vi "ModemTelemetryDecode.vi"(8 "Error In":errorcluster, 11 "Encoded Data":u8[](array[numeric])) -> (0 "Error Out":errorcluster, 3 "TelemetryPacket":T1)   [LabVIEW 2010]
uses:
  ModemTelemetryPacket.ctl
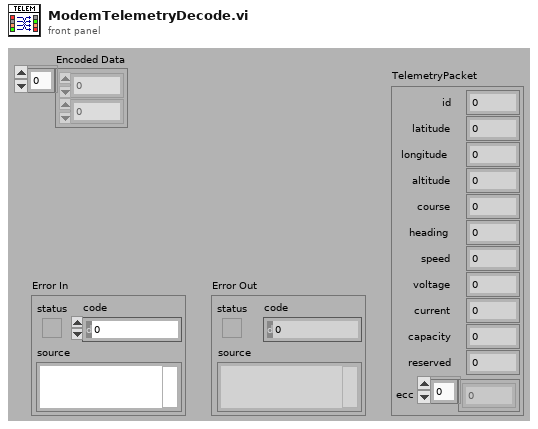
[diagram p1: front panel]
types:
  T1 = typedef "ModemTelemetryPacket.ctl" = cluster{"id":u16, "latitude":i32, "longitude":i32, "altitude":i16, "course":i16, "heading":i16, "speed":i16, "voltage":u8, "current":u8, "capacity":u16, "reserved":u16, "ecc":u8[]}
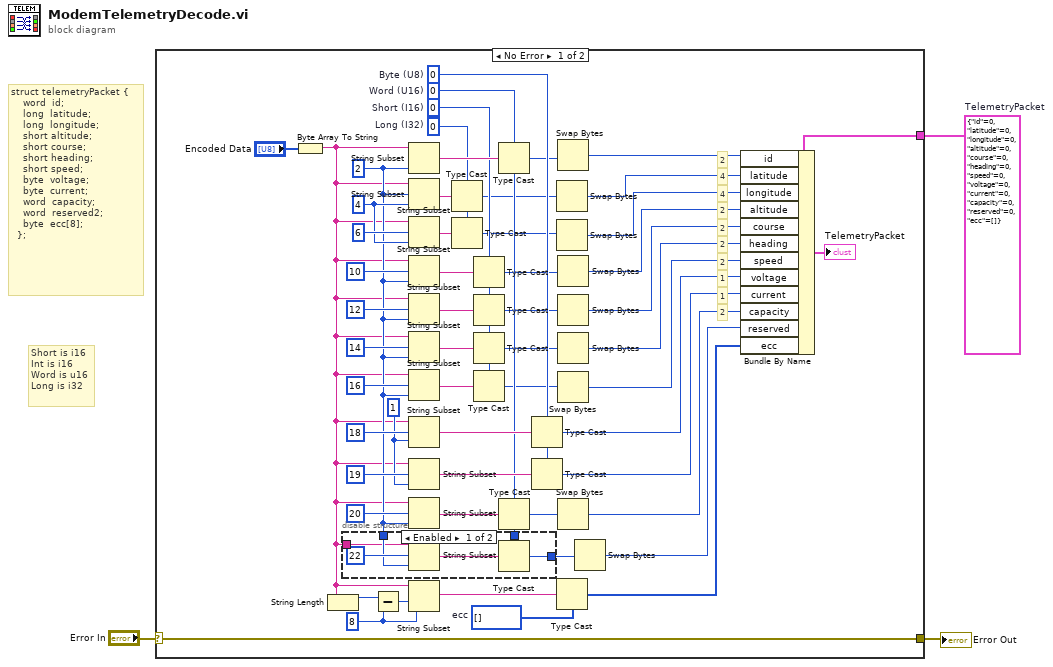
[diagram p0: block diagram]
diagram:
  w1 = T1 {"id"=0, "latitude"=0, "longitude"=0, "altitude"=0, "course"=0, "heading"=0, "speed"=0, "voltage"=0, "current"=0, "capacity"=0, "reserved"=0, "ecc"=[]}  # TelemetryPacket
  # "struct telemetryPacket {\n    word  id;\n    long  latitude;\n    long  longitude;\n    short altitude;\n    short course;\n    short heading;\n    short speed;\n    byte  voltage;\n    byte  current;\n    word  capacity;\n    word  reserved2;\n    byte  ecc[8];\n  };"
  # "Short is i16\nInt is i16\nWord is u16\nLong is i32"
  n1 = case shown="No Error" "Error In" {
    selector: "Error In" -> [w59 w66]
    tunnel: [w59 w66] -> w2
    tunnel: w1 -> [w57 _]
    frame No Error {
      w22 = u16 0  # Word (U16)
      w24 = 8 ("length (rest)")
      w29 = u8[] []  # ecc
      w36 = 1 ("length (rest)")
      w37 = u8 0  # Byte (U8)
      w52 = 0  # Long (I32)
      w49 = 4 ("length (rest)")
      w23 = i16 0  # Short (I16)
      w31 = 2 ("length (rest)")
      # "2"
      # "1"
      # "1"
      # "2"
      # "2"
      # "2"
      # "2"
      # "4"
      # "4"
      # "2"
      n2 = Byte Array To String(unsigned byte array="Encoded Data") -> (string=w27:string)
      n3 = String Length(string=w27) -> (length=w26:i32)
      n4 = disable-structure shown="Enabled" {
        disable-tunnel: w31 -> [w64 _]
        disable-tunnel: [w63 _] -> w12
        disable-tunnel: w22 -> [w62 _]
        disable-tunnel: w27 -> [w60 _]
        frame Enabled {
          n5 = String Subset(string=w60, offset (0)=22, length (rest)=w64) -> (substring=w61:string)
          n6 = Type Cast(type=w62, x=w61) -> (*(type *) &x=w63:u16)
        }
        frame Disabled {
          # "No Used For Now"
        }
      }
      n7 = Subtract(x=w26, y=w24) -> (x-y=w25:i32)
      n8 = String Subset(string=w27, length (rest)=w31) -> (substring=w55:string)  [unwired: 1 in]
      n9 = String Subset(string=w27, offset (0)=w31, length (rest)=w49) -> (substring=w54:string)
      n10 = String Subset(string=w27, offset (0)=6, length (rest)=w49) -> (substring=w50:string)
      n11 = String Subset(string=w27, offset (0)=10, length (rest)=w31) -> (substring=w47:string)
      n12 = String Subset(string=w27, offset (0)=12, length (rest)=w31) -> (substring=w44:string)
      n13 = String Subset(string=w27, offset (0)=14, length (rest)=w31) -> (substring=w46:string)
      n14 = String Subset(string=w27, offset (0)=16, length (rest)=w31) -> (substring=w41:string)
      n15 = String Subset(string=w27, offset (0)=18, length (rest)=w36) -> (substring=w40:string)
      n16 = String Subset(string=w27, offset (0)=19, length (rest)=w36) -> (substring=w33:string)
      n17 = String Subset(string=w27, offset (0)=20, length (rest)=w31) -> (substring=w32:string)
      n18 = String Subset(string=w27, offset (0)=w25, length (rest)=w24) -> (substring=w30:string)
      n19 = Type Cast(type=w52, x=w54) -> (*(type *) &x=w9:i32)
      n20 = Type Cast(type=w52, x=w50) -> (*(type *) &x=w8:i32)
      n21 = Type Cast(type=w23, x=w47) -> (*(type *) &x=w21:i16)
      n22 = Type Cast(type=w23, x=w44) -> (*(type *) &x=w5:i16)
      n23 = Type Cast(type=w23, x=w46) -> (*(type *) &x=w18:i16)
      n24 = Type Cast(type=w23, x=w41) -> (*(type *) &x=w16:i16)
      n25 = Type Cast(type=w22, x=w55) -> (*(type *) &x=w19:u16)
      n26 = Type Cast(type=w22, x=w32) -> (*(type *) &x=w14:u16)
      n27 = Type Cast(type=w37, x=w40) -> (*(type *) &x=w38:u8)
      n28 = Type Cast(type=w37, x=w33) -> (*(type *) &x=w35:u8)
      n29 = Swap Bytes(anything=w9) -> (byte swapped=w7:i32)
      n30 = Swap Bytes(anything=w8) -> (byte swapped=w6:i32)
      n31 = Type Cast(type=w29, x=w30) -> (*(type *) &x=w28:u8[])
      n32 = Swap Bytes(anything=w19) -> (byte swapped=w10:u16)
      n33 = Swap Bytes(anything=w21) -> (byte swapped=w20:i16)
      n34 = Swap Bytes(anything=w5) -> (byte swapped=w4:i16)
      n35 = Swap Bytes(anything=w18) -> (byte swapped=w17:i16)
      n36 = Swap Bytes(anything=w16) -> (byte swapped=w15:i16)
      n37 = Swap Bytes(anything=w14) -> (byte swapped=w13:u16)
      n38 = Swap Bytes(anything=w12) -> (byte swapped=w11:u16)
      n39 = Bundle By Name(cluster=w57, "id"=w10, "latitude"=w7, "longitude"=w6, "altitude"=w20, "course"=w4, "heading"=w17, "speed"=w15, "voltage"=w38, "current"=w35, "capacity"=w13, "reserved"=w11, "ecc"=w28) -> (→"TelemetryPacket":T1)
    }
    frame Error {
    }
  }
  "Error Out" <- w2
